vi "Error From Code.vi"(8 "error in (no error)":errorcluster, 11 "ErrorCode":i32) -> (0 "error out":errorcluster)   [LabVIEW 2013, in "Capacitive.lvlib"]
uses:
  Capacitive.lvlib
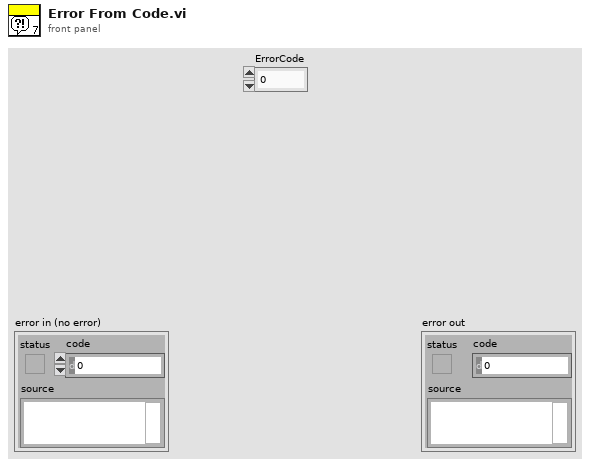
[diagram p1: front panel]
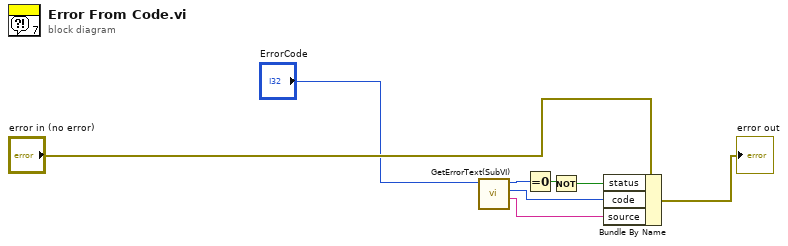
[diagram p0: block diagram]
diagram:
  n1 = call "GetErrorText(SubVI).vi"("ErrorCode"="ErrorCode") -> ("ErrorText"=w4:string, "ErrorCode"=w5:i32, "Status"=w8:i32)  [unwired: 8 in]
  n2 = Equal To 0?(x=w8) -> (x = 0?=w7:bool)
  n3 = Not(x=w7) -> (.not. x?=w6:bool)
  n4 = Bundle By Name(cluster="error in (no error)", "status"=w6, "code"=w5, "source"=w4) -> (→"error out":errorcluster)
